vi "Set PID.vi"(8 "error in (no error)":errorcluster, 10 "PID":T1, 11 "PIDController in":refnum<class "PIDController.lvclass">) -> (0 "error out":errorcluster, 3 "PIDController out":refnum<class "PIDController.lvclass">)   [LabVIEW 2023, in "PIDController.lvclass"]
uses:
  PIDController.lvclass
  PIDController.lvclass/PIDController.ctl
  PIDModBus/Controls/PID Cluster.ctl
  PIDModBus/PIDModbus.lvlib
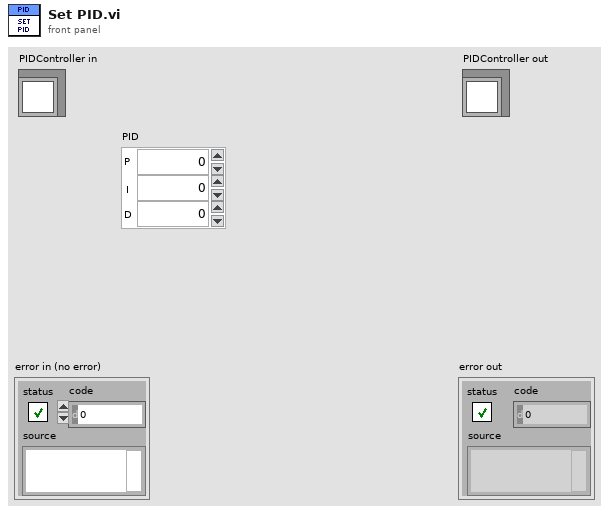
[diagram p1: front panel]
types:
  T1 = typedef "PIDModbus.lvlib/PID Cluster.ctl" = cluster{"P":u16, "I":u16, "D":u16}
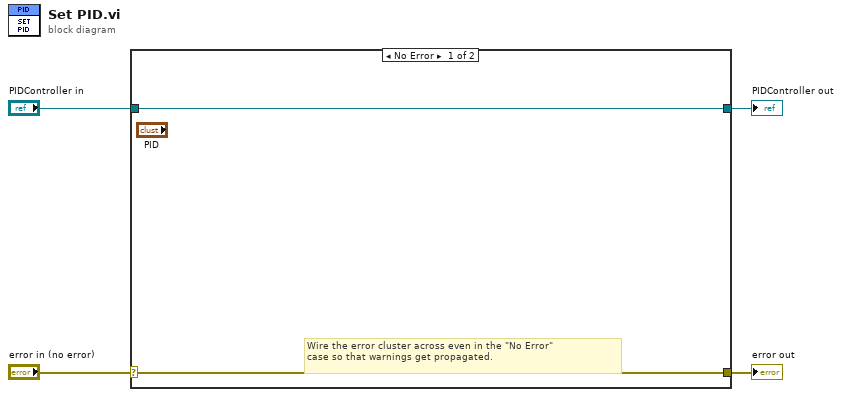
[diagram p0: block diagram]
diagram:
  n1 = case shown="No Error" "error in (no error)" {
    selector: "error in (no error)" -> [w5 w8]
    tunnel: [w5 w8] -> w3
    tunnel: [w6 w7] -> w1
    tunnel: "PIDController in" -> [w6 w7]
    frame No Error {
      # "Wire the error cluster across even in the \"No Error\"\ncase so that warnings get propagated."
    }
    frame Error {
    }
  }
  "error out" <- w3
  "PIDController out" <- w1
